vi "Run VI from Methods Folder.vi"(7 "Request":refnum<class "Request.lvclass">, 8 "error in (no error)":errorcluster, 9 "JSON Value in":refnum<class "JSON Value.lvclass">, 10 "String":string, 11 "JSONRPC Server in":refnum<class "JSONRPC Server.lvclass">) -> (0 "error out":errorcluster, 3 "JSONRPC Server out":refnum<class "JSONRPC Server.lvclass">)   [LabVIEW 2016]
uses:
  JSONRPC Server.lvclass
  Add Response (Result from Request).vi
  Add Response (Internal Error from Request).vi
  Add Response (Method Not Found from Request).vi
  <vilib>/NI/JSON Support for LabVIEW/JSON Value/JSON Value.lvclass
  <vilib>/NI/JSON Support for LabVIEW/JSON Value/New JSON Value/New JSON (String).vi
  Request/Request.lvclass
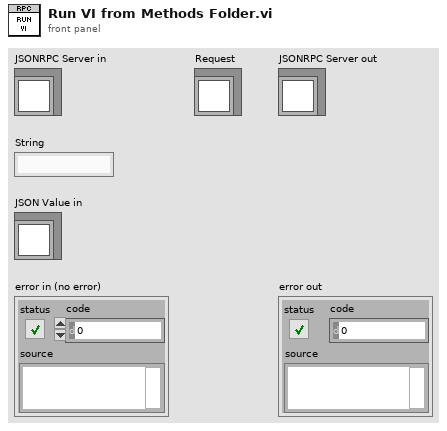
[diagram p1: front panel]
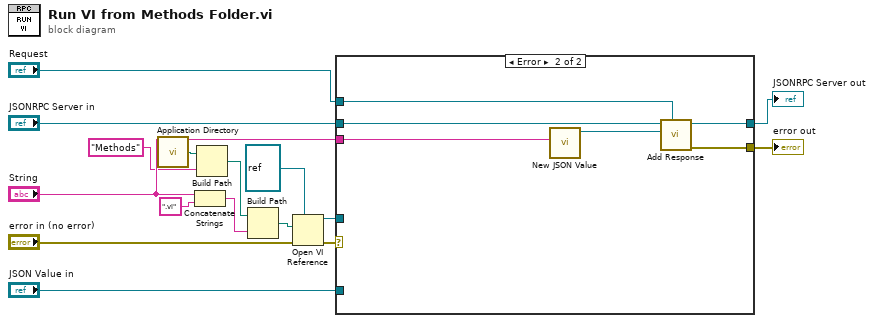
[diagram p0: block diagram]
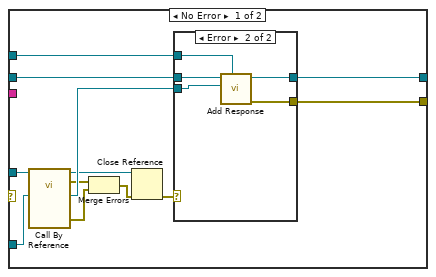
[diagram p2: hidden frame]
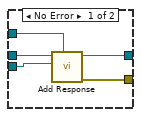
[diagram p3: hidden frame]
diagram:
  n1 = call <vilib>:"Application Directory.vi"() -> ("Application Directory"=w4:path)
  n2 = Concatenate Strings("String", ".vi" ("string")) -> (w9:string)
  n3 = Build Path(base path=w4, name or relative path="Methods") -> (appended path=w2:path)
  n4 = Build Path(base path=w2, name or relative path=w9) -> (appended path=w8:path)
  n5 = Open VI Reference(type specifier VI Refnum (for type only)=refnum<vi> refnum, vi path=w8, error in (no error)="error in (no error)") -> (vi reference=w6:refnum<vi>, error out=w7:errorcluster)  [unwired: 3 in]
  n6 = case shown="Error" w7 {
    tunnel: "JSONRPC Server in" -> [w28 w43]
    tunnel: "Request" -> [w27 w44]
    tunnel: [w26 w41] -> w15
    tunnel: [w25 w42] -> w16
    tunnel: w6 -> [w24 _]
    tunnel: "JSON Value in" -> [w23 _]
    tunnel: "String" -> [_ w40]
    frame No Error {
      n7 = call-by-ref "?"(reference=w24, "params"=w23) -> (reference out=w18:refnum<vi>, error out=w21:errorcluster, 0:"error out"=w20:errorcluster, "data"=w22:refnum<class "JSON Value.lvclass">)  [unwired: 10 in]
      n8 = Merge Errors(w21, w20) -> (w19:errorcluster)
      n9 = Close Reference(reference=w18, error in (no error)=w19) -> (error out=w17:errorcluster)
      n10 = case shown="Error" w17 {
        tunnel: w28 -> [w33 w38]
        tunnel: w27 -> [w32 w37]
        tunnel: [w31 w36] -> w26
        tunnel: [w30 w35] -> w25
        tunnel: w22 -> [w29 w34]
        frame No Error {
          n11 = call-poly "Add Response.vi"("Request"=w32, "JSON Value in"=w29, "Server in"=w33) -> ("error out"=w31:errorcluster, "Server out"=w30:refnum<class "JSONRPC Server.lvclass">)  [unwired: 6 in, 1 out]
        }
        frame Error {
          n12 = call-poly "Add Response.vi"("Request"=w37, "data"=w34, "Server in"=w38) -> ("error out"=w36:errorcluster, "Server out"=w35:refnum<class "JSONRPC Server.lvclass">)  [unwired: 6 in, 1 out]
        }
      }
    }
    frame Error {
      n13 = call-poly <vilib>:"New JSON Value.vi"("value"=w40) -> ("JSON Value out"=w39:refnum<class "JSON Value.lvclass">)  [unwired: 9 in, 1 out]
      n14 = call-poly "Add Response.vi"("Request"=w44, "data"=w39, "Server in"=w43) -> ("error out"=w41:errorcluster, "Server out"=w42:refnum<class "JSONRPC Server.lvclass">)  [unwired: 6 in, 1 out]
    }
  }
  "JSONRPC Server out" <- w16
  "error out" <- w15
